vi "tsapp_set_canlin_channel_count_win32.vi"(8 "错误输入（无错误）":errorcluster, 10 "InitializationInformation":T1 {"LIN使用通道数" max=5; "CAN使用通道数" max=5}) -> (0 "错误输出":errorcluster, 1 "InitializationInformation_Out":T1 {"LIN使用通道数" max=5; "CAN使用通道数" max=5}, 2 "SetSuccessfully":bool)   [LabVIEW 2016]
uses:
  CAN_Info.ctl
  D:/Program Files (x86)/TOSUN/TSMaster/bin/Data/SDK/lib/x86/TSMaster.dll
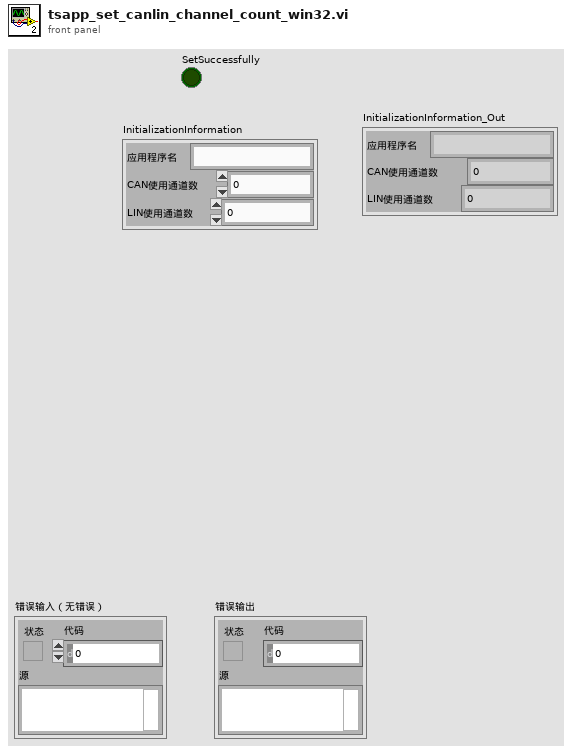
[diagram p1: front panel]
types:
  T1 = typedef "CAN_Info.ctl" = cluster{"应用程序名":string, "CAN使用通道数":u8, "LIN使用通道数":u8}
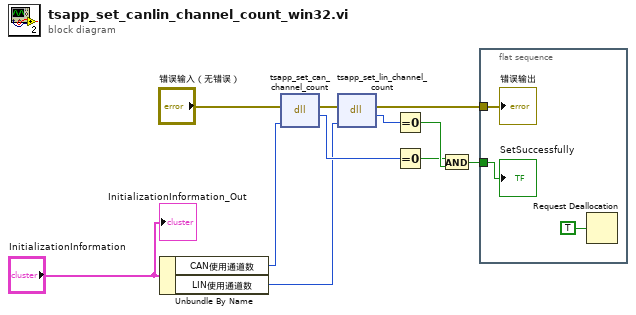
[diagram p0: block diagram]
diagram:
  n1 = Unbundle By Name("InitializationInformation") -> ("CAN使用通道数"=w4:u8, "LIN使用通道数"=w6:u8)
  n2 = dll-call lib="D:/Program Files (x86)/TOSUN/TSMaster/bin/Data/SDK/lib/x86/TSMaster.dll" fn="tsapp_set_can_channel_count"(error in="错误输入（无错误）", "ACount"=w4) -> (error out=w1:errorcluster, "tsapp_set_can_channel_count"=w10:i32)  [unwired: 3 in, 1 out]
  n3 = dll-call lib="D:/Program Files (x86)/TOSUN/TSMaster/bin/Data/SDK/lib/x86/TSMaster.dll" fn="tsapp_set_lin_channel_count"(error in=w1, "ACount"=w6) -> (error out=w5:errorcluster, "tsapp_set_can_channel_count"=w2:i32)  [unwired: 3 in, 1 out]
  n4 = Equal To 0?(x=w2) -> (x = 0?=w9:bool)
  n5 = Equal To 0?(x=w10) -> (x = 0?=w8:bool)
  n6 = And(x=w8, y=w9) -> (x .and. y?=w11:bool)
  n7 = flat-sequence {
    tunnel: w11 -> [w14]
    tunnel: w5 -> [w13]
    frame #0 {
      n8 = Request Deallocation(TRUE ("标志")) -> ()
      "SetSuccessfully" <- w14
      "错误输出" <- w13
    }
  }
  "InitializationInformation_Out" <- "InitializationInformation"
